vi "TDMS GET DATA G3.vi"(7 "OffSet In":i64, 8 "error in":errorcluster, 10 "max":i64, 11 "tdms file In":refnum<k34>) -> (0 "error out 2":errorcluster, 3 "Result":T1(array[cluster]), 4 "lengh":i64, 5 "Repetir":bool)   [LabVIEW 2015]
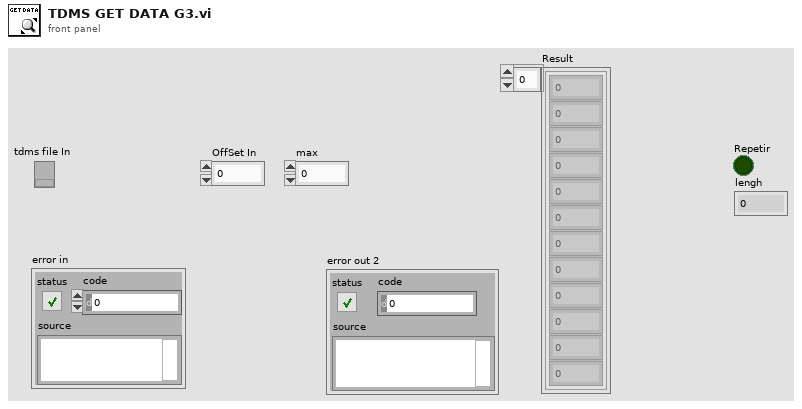
[diagram p1: front panel]
types:
  T1 = cluster{u32, dbl, dbl, dbl, dbl, dbl, dbl, dbl, dbl, dbl, dbl, dbl}[]
  T2 = cluster{u32, dbl, dbl, dbl, dbl, dbl, dbl, dbl, dbl, dbl, dbl, dbl}
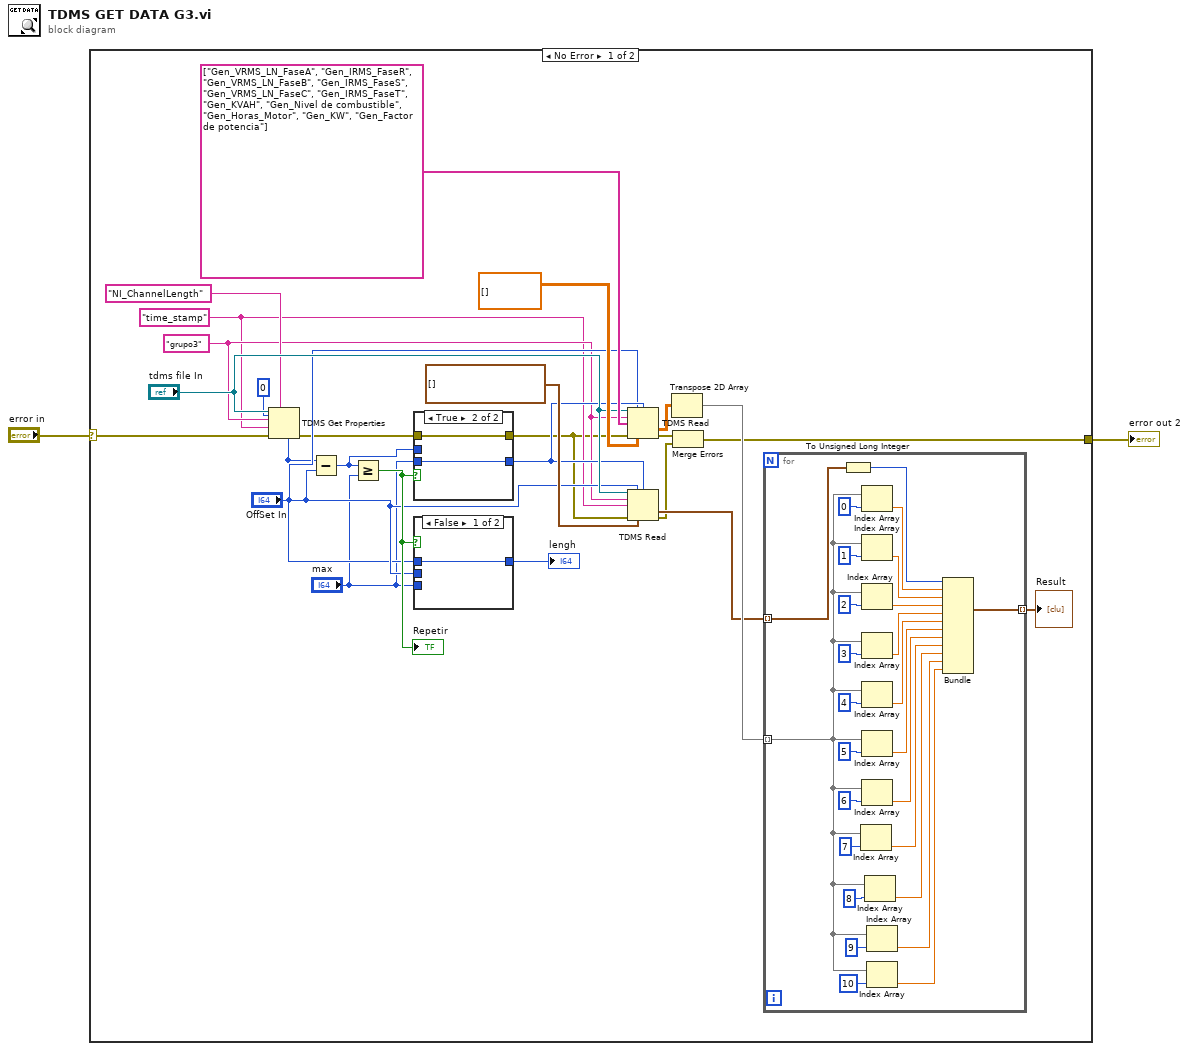
[diagram p0: block diagram]
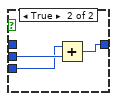
[diagram p2: hidden frame]
diagram:
  n1 = case shown="No Error" "error in" {
    selector: "error in" -> [w5 w62]
    tunnel: [w18 w62] -> w2
    frame No Error {
      w10 = "time_stamp"
      w11 = "grupo3"
      n2 = TDMS Get Properties(5:i64 0, 7:"NI_ChannelLength" ("property name"), 8:w5, 9:w10, 10:w11, 11:"tdms file In") -> (0:w9:errorcluster, 4:w13:i64)  [unwired: 4 out]
      n3 = Subtract(x=w13, y="OffSet In") -> (x-y=w17:i64)
      n4 = Greater Or Equal?(x=w17, y="max") -> (x >= y?=w15:bool)
      "Repetir" <- w15
      n5 = case shown="True" w15 {
        tunnel: [w33 w34] -> w16
        tunnel: w17 -> [w33 _]
        tunnel: w9 -> [w32 w35]
        tunnel: [w32 w35] -> w8
        tunnel: "max" -> [_ w34]
        frame False {
        }
        frame True {
        }
      }
      n6 = case shown="False" w15 {
        tunnel: "OffSet In" -> [_ w31]
        tunnel: [w28 w30] -> w12
        tunnel: w13 -> [w28 _]
        tunnel: "max" -> [_ w29]
        frame False {
        }
        frame True {
          n7 = Add(x=w29, y=w31) -> (x+y=w30:i64)
        }
      }
      "lengh" <- w12
      n8 = TDMS Read(0:"tdms file In", 1:"OffSet In", 2:w16, 5:w11, 7:string[] ["Gen_VRMS_LN_FaseA", "Gen_IRMS_FaseR", "Gen_VRMS_LN_FaseB", "Gen_IRMS_FaseS", "Gen_VRMS_LN_FaseC", "Gen_IRMS_FaseT", "Gen_KVAH", "Gen_Nivel de combustible", "Gen_Horas_Motor", "Gen_KW", "Gen_Factor de potencia"], 11:w8, 12:dbl[][] []) -> (10:w25:dbl[][], 15:w19:errorcluster)  [unwired: 1 in, 4 out]
      n9 = TDMS Read(0:"tdms file In", 1:"OffSet In", 2:w16, 5:w11, 7:w10, 11:w8, 12:timestamp[] []) -> (10:w6:timestamp[], 15:w4:errorcluster)  [unwired: 1 in, 4 out]
      n10 = Transpose 2D Array(2D array=w25) -> (transposed array=w24:dbl[][])
      n11 = Merge Errors(w19, w4) -> (w18:errorcluster)
      n12 = for {
        tunnel: w6 -> [w61] mode=indexing
        tunnel: w24 -> [w38] mode=indexing
        tunnel: [w51] -> w3 mode=indexing
        n13 = To Unsigned Long Integer(number=w61) -> (unsigned 32bit integer=w56:u32)
        n14 = Index Array(array=w38, index=7) -> (element=w43:dbl)
        n15 = Index Array(array=w38, index=0) -> (element=w55:dbl)
        n16 = Index Array(array=w38, index=1) -> (element=w54:dbl)
        n17 = Index Array(array=w38, index=2) -> (element=w53:dbl)
        n18 = Index Array(array=w38, index=3) -> (element=w52:dbl)
        n19 = Index Array(array=w38, index=4) -> (element=w49:dbl)
        n20 = Index Array(array=w38, index=5) -> (element=w47:dbl)
        n21 = Index Array(array=w38, index=6) -> (element=w45:dbl)
        n22 = Index Array(array=w38, index=8) -> (element=w41:dbl)
        n23 = Index Array(array=w38, index=9) -> (element=w39:dbl)
        n24 = Index Array(array=w38, index=10) -> (element=w36:dbl)
        n25 = Bundle(w56, w55, w54, w53, w52, w49, w47, w45, w43, w41, w39, w36) -> (w51:T2)  [unwired: 1 in]
      }
      "Result" <- w3
    }
    frame Error {
    }
  }
  "error out 2" <- w2
